vi "mcl_move_piezos.vi"(8 "error in (no error)":errorcluster, 10 "new_positions":dbl[](array[numeric]), 11 "thorlabs_panel in":refnum<class "mcl_panel.lvclass">) -> (0 "error out":errorcluster, 3 "thorlabs_panel out":refnum<class "mcl_panel.lvclass">)   [LabVIEW 2015, in "mcl_panel.lvclass"]
uses:
  mcl_panel.lvclass
  mcl_piezo_class/mcl_piezo.lvclass
  UI/panel_class/panel.lvclass
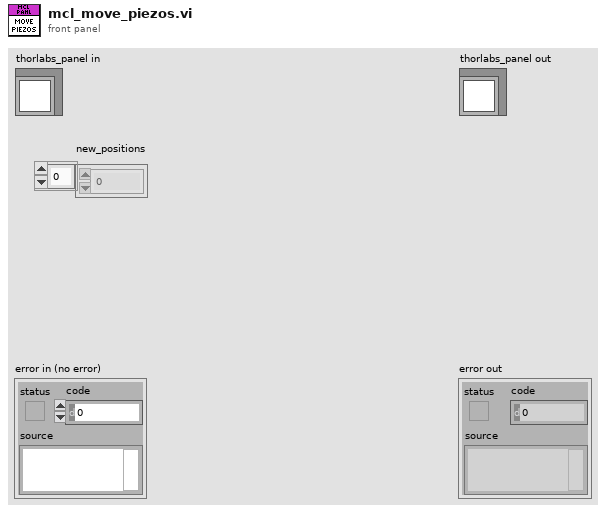
[diagram p1: front panel]
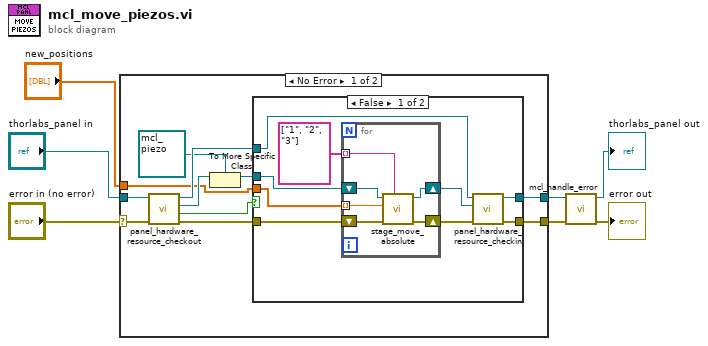
[diagram p0: block diagram]
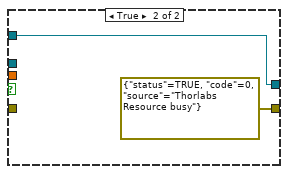
[diagram p2: hidden frame]
diagram:
  n1 = case shown="No Error" "error in (no error)" {
    selector: "error in (no error)" -> [w17 w37]
    tunnel: [w10 w37] -> w1
    tunnel: [w9 w36] -> w4
    tunnel: "thorlabs_panel in" -> [w18 w36]
    tunnel: "new_positions" -> [w11 _]
    frame No Error {
      n2 = call "panel_hardware_resource_checkout.vi"("error in (no error)"=w17, "panel in"=w18) -> ("error out"=w14:errorcluster, "timed out?"=w13:bool, "hardware.lvclass"=w16:refnum<class "hardware.lvclass">, "panel out"=w12:refnum<class "mcl_panel.lvclass">)  [unwired: 6 in]
      n3 = To More Specific Class(target class=refnum<class "mcl_piezo.lvclass"> refnum ("mcl_piezo.lvclass"), reference=w16) -> (specific class reference=w15:refnum<class "mcl_piezo.lvclass">)  [unwired: 1 in, 1 out]
      n4 = case shown="False" w13 {
        tunnel: w15 -> [w22 _]
        tunnel: w14 -> [w23 _]
        tunnel: w12 -> [w25 w34]
        tunnel: [w27 w34] -> w9
        tunnel: [w26 errorcluster {"status"=TRUE, "code"=0, "source"="Thorlabs Resource busy"} ("error out")] -> w10
        tunnel: w11 -> [w24 _]
        frame False {
          n5 = for {
            tunnel: w24 -> [w29] mode=indexing
            shift-right: [w31] -> w21
            shift-left: w23 -> [w30]
            shift-right: [w32] -> w20
            shift-left: w22 -> [w33]
            tunnel: string[] ["1", "2", "3"] -> [w28] mode=indexing
            n6 = call-dynamic "stage_move_absolute.vi"("Stage Name"=w28, "error in (no error)"=w30, "Position"=w29, "mcl_piezo in"=w33) -> ("error out"=w31:errorcluster, "mcl_piezo out"=w32:refnum<class "mcl_piezo.lvclass">)  [unwired: 6 in]
          }
          n7 = call "panel_hardware_resource_checkin.vi"("error in (no error)"=w21, "hardware.lvclass"=w20, "panel in"=w25) -> ("error out"=w26:errorcluster, "panel out"=w27:refnum<class "mcl_panel.lvclass">)  [unwired: 7 in]
        }
        frame True {
        }
      }
    }
    frame Error {
    }
  }
  n8 = call "mcl_handle_error.vi"("error in (no error)"=w1, "thorlabs_panel in"=w4) -> ("error out"=→"error out":errorcluster, "thorlabs_panel out"=→"thorlabs_panel out":refnum<class "mcl_panel.lvclass">)  [unwired: 8 in]
